vi "Quick Analog Input.vi"() -> ()   [LabVIEW 2020]
panel:
  out "Array":dbl[](array[numeric])
  in  "stop":bool
  out "Waveform Graph":dbl[](graph)
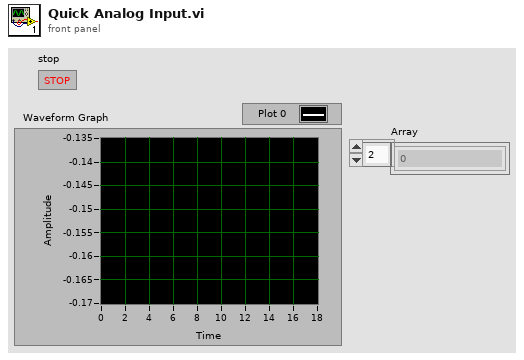
[diagram p1: front panel]
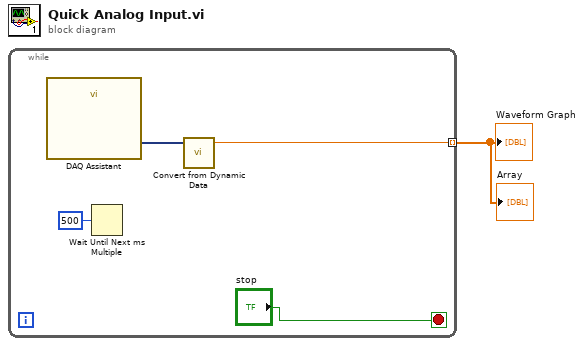
[diagram p0: block diagram]
diagram:
  n1 = while {
    tunnel: [w2] -> w1 mode=indexing
    stop <- "stop" stop-if-true
    n2 = call "DAQ Assistant"() -> ("data"=w3:dynamicdata)  [unwired: 17 in, 2 out]
    n3 = Wait Until Next ms Multiple(millisecond multiple=u32 500) -> ()  [unwired: 1 out]
    n4 = call "Convert from Dynamic Data"("Dynamic Data Type"=w3) -> ("Scalar"=w2:dbl)  [unwired: 3 in]
  }
  "Waveform Graph" <- w1
  "Array" <- w1
